vi "InterpSecImage.vi"() -> ()   [LabVIEW 2022 SP3]
panel:
  in  "Save Interp Image?":bool
  out "Raw data":i16[][](graph)
  in  "reduce pts by factor of":i32=1
  in  "PTs on Axis":u16[](array[numeric])
  in  "Choose Pts\non Axis?":bool
  out "Interpolated Sector Intensity Graph":i16[][](graph)
  out "# lines per scan":u16
  out "# rf points per line":u16
  out "sector scan angle":sgl format="%.2f"
  in  "new file path":path=path "C:/WINDOWS/DESKTOP/Q140r18.eye"
  out "z":i8[][](array[numeric])
  out "y":dbl[][](array[numeric]) format="%.4f"
  out "x":dbl[][](array[numeric]) format="%.5f"
  in  "Read File?":bool
  # "© 2000 Riverside Research Institute"
  # "rows"
  # "columns"
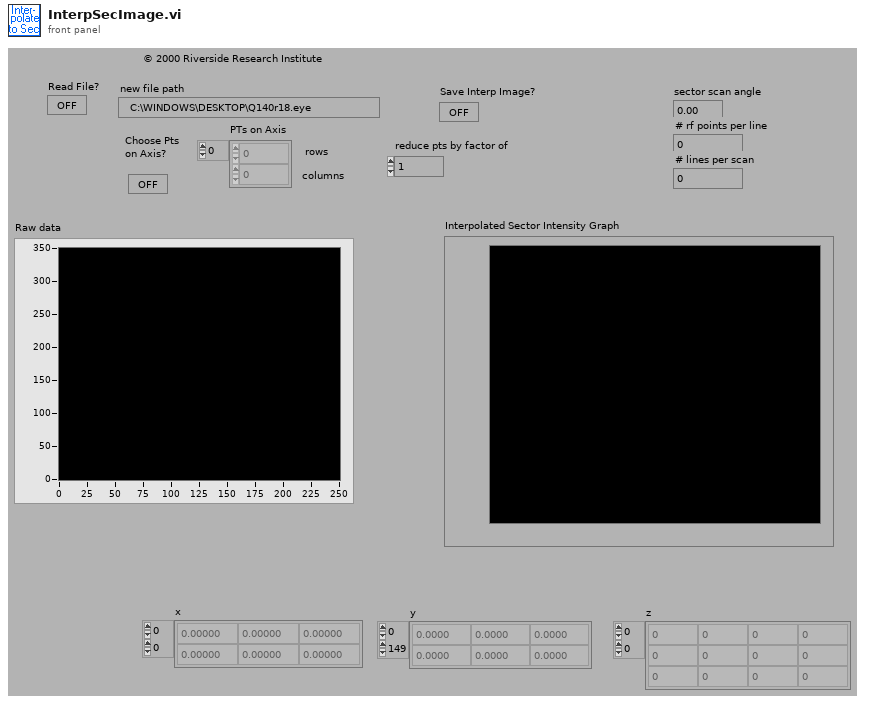
[diagram p1: front panel]
types:
  T1 = cluster{"delay":sgl, "pivot distance":sgl, "sector scan angle":sgl, "operator":string, "Scan Mode":string, "location":string}
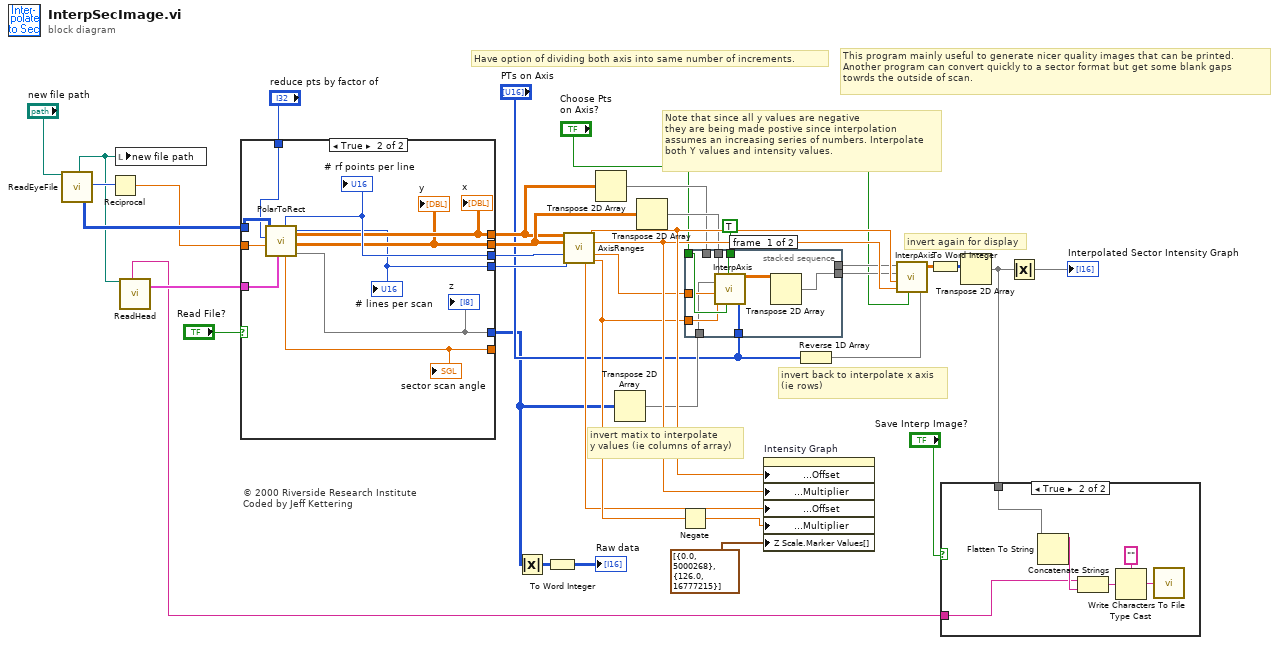
[diagram p0: block diagram]
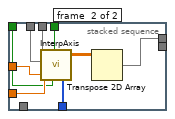
[diagram p3: hidden frame]
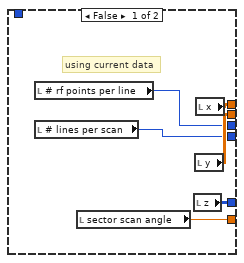
[diagram p4: hidden frame]
diagram:
  # "© 2000 Riverside Research Institute\nCoded by Jeff Kettering"
  # "This program mainly useful to generate nicer quality images that can be printed.\nAnother program can convert quickly to a sector format but get some blank gaps\ntowrds the outside of scan."
  # "Have option of dividing both axis into same number of increments."
  # "invert again for display"
  # "invert back to interpolate x axis \n(ie rows)"
  # "invert matix to interpolate \ny values (ie columns of array)"
  # "Note that since all y values are negative\nthey are being made postive since interpolation \nassumes an increasing series of numbers. Interpolate\nboth Y values and intensity values."
  n1 = call "ReadEyeFile.vi"("new file path"="new file path") -> ("new path out"=w5:path, "2-D data array"=w9:i16[][], "sample rate MHz"=w8:u16)  [unwired: 1 in, 15 out]
  n2 = Reciprocal(x=w8) -> (1/x=w7:dbl)
  n3 = local write "new file path"(w5) -> ()
  n4 = call "ReadHead.vi"("new file path"=w5) -> ("whole header"=w2:string, "Scan Info"=w6:T1)  [unwired: 17 out]
  n5 = case shown="True" "Read File?" {
    tunnel: [w41 w51] -> w25
    tunnel: [w42 w50] -> w34
    tunnel: [w43 w48] -> w14
    tunnel: [w40 w53] -> _
    tunnel: [w39 w49] -> w35
    tunnel: [w38 w52] -> w36
    tunnel: "reduce pts by factor of" -> [_ w46]
    tunnel: w9 -> [_ w47]
    tunnel: w7 -> [_ w45]
    tunnel: w6 -> [_ w44]
    frame False {
      # "using current data"
      n6 = local read "# rf points per line"() -> (w38:u16)
      n7 = local read "# lines per scan"() -> (w39:u16)
      n8 = local read "sector scan angle"() -> (w40:sgl)
      n9 = local read "z"() -> (w43:i8[][])
      n10 = local read "y"() -> (w42:dbl[][])
      n11 = local read "x"() -> (w41:dbl[][])
    }
    frame True {
      n12 = call "PolarToRect.vi"("Scan Info"=w44, "Time between pt\nmicros"=w45, "c m/s"=w46, "array dims"=w47) -> (0:w48, "y"=w50:dbl[][], "x"=w51:dbl[][], "# lines per scan"=w49:u16, "sector scan angle"=w53:sgl, "# rf points per line"=w52:u16)  [unwired: 2 out]
      "x" <- w51
      "y" <- w50
      "z" <- w48
      "sector scan angle" <- w53
      "# rf points per line" <- w52
      "# lines per scan" <- w49
    }
  }
  n13 = Absolute Value(x=w14) -> (abs(x)=w13:i8[][])
  n14 = To Word Integer(number=w13) -> (16bit integer=→"Raw data":i16[][])
  n15 = call "AxisRanges.vi"("x"=w25, "y"=w34, "# rf points per line"=w36, "# lines per scan"=w35) -> ("X left"=w33:dbl, "X step"=w32:dbl, "Y low"=w30:dbl, "Y high"=w29:dbl, "Y step"=w31:dbl)  [unwired: 2 in, 5 out]
  n16 = Transpose 2D Array(2D array=w25) -> (transposed array=w22:dbl[][])
  n17 = Transpose 2D Array(2D array=w14) -> (transposed array=w27:i8[][])
  n18 = Transpose 2D Array(2D array=w34) -> (transposed array=w24:dbl[][])
  n19 = Negate(x=w31) -> (-x=w28:dbl)
  n20 = stacked-sequence {
    tunnel: "Choose Pts\non Axis?" -> [w62 w68]
    tunnel: "PTs on Axis" -> [w61 w63]
    tunnel: w31 -> [w60 w69]
    tunnel: w30 -> [w59 w70]
    tunnel: w27 -> [w58 _]
    tunnel: TRUE ("Invert Y ?") -> [w57 w71]
    tunnel: w24 -> [w55 w67]
    tunnel: [w54 _] -> w23
    tunnel: w22 -> [_ w66]
    tunnel: [_ w64] -> w21
    frame #0 {
      n21 = call "InterpAxis.vi"("co-ord array"=w55, "Invert Y ?"=w57, "z in"=w58, "start value"=w59, "Choose Pts?"=w62, "step size"=w60, "PTs on Axis"=w61) -> ("z interp"=w56:dbl[][])  [unwired: 1 out]
      n22 = Transpose 2D Array(2D array=w56) -> (transposed array=w54:dbl[][])
    }
    frame #1 {
      n23 = call "InterpAxis.vi"("co-ord array"=w67, "Invert Y ?"=w71, "z in"=w66, "start value"=w70, "Choose Pts?"=w68, "step size"=w69, "PTs on Axis"=w63) -> ("z interp"=w65:dbl[][])  [unwired: 1 out]
      n24 = Transpose 2D Array(2D array=w65) -> (transposed array=w64:dbl[][])
    }
  }
  n25 = property on="Intensity Graph" class="IntGraph (strict)"("X Scale.Offset and Multiplier:Offset"=w33, "X Scale.Offset and Multiplier:Multiplier"=w32, "Y Scale.Offset and Multiplier:Offset"=w29, "Y Scale.Offset and Multiplier:Multiplier"=w28, "Z Scale.Marker Values[]"=cluster{dbl, u32}[] [{0.0, 5000268}, {126.0, 16777215}] ("color scheme 3")) -> ()  [unwired: 2 in, 2 out]
  n26 = Reverse 1D Array(array="PTs on Axis") -> (reversed array=w20:u16[])
  n27 = call "InterpAxis.vi"("co-ord array"=w21, "z in"=w23, "start value"=w33, "Choose Pts?"="Choose Pts\non Axis?", "step size"=w32, "PTs on Axis"=w20) -> ("z interp"=w18:dbl[][])  [unwired: 1 in, 1 out]
  n28 = To Word Integer(number=w18) -> (16bit integer=w11:i16[][])
  n29 = Transpose 2D Array(2D array=w11) -> (transposed array=w17:i16[][])
  n30 = case shown="True" "Save Interp Image?" {
    tunnel: w17 -> [_ w73]
    tunnel: w2 -> [_ w72]
    frame False {
    }
    frame True {
      n31 = Flatten To String(anything=w73) -> (data string=w76:string)  [unwired: 1 in, 4 out]
      n32 = Concatenate Strings(w72, w76) -> (w74:string)
      n33 = Type Cast(type="", x=w74) -> (*(type *) &x=w75:string)
      n34 = call <vilib>:"Write Characters To File.vi"("character string"=w75) -> ()  [unwired: 2 in, 3 out]
    }
  }
  n35 = Absolute Value(x=w17) -> (abs(x)=→"Interpolated Sector Intensity Graph":i16[][])
